vi "Generate GUID.vi"(8 "error in (no error)":errorcluster) -> (0 "error out":errorcluster, 3 "GUID":string)   [LabVIEW 2014]
panel:
  in  ".NET Refnum":refnum<k24>
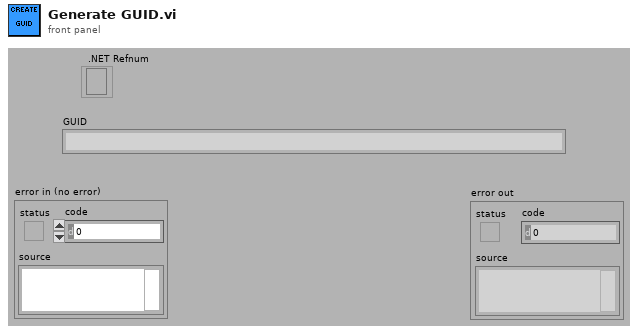
[diagram p1: front panel]
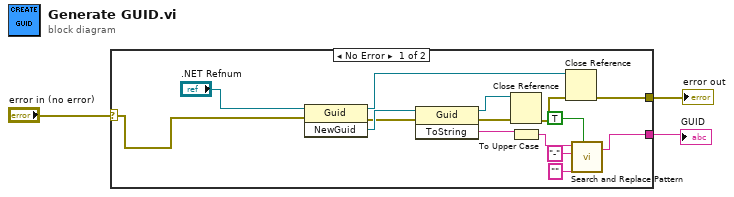
[diagram p0: block diagram]
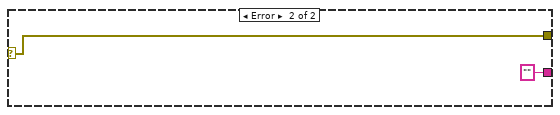
[diagram p2: hidden frame]
diagram:
  n1 = case shown="No Error" "error in (no error)" {
    selector: "error in (no error)" -> [w4 w20]
    tunnel: [w14 w20] -> w2
    tunnel: [w7 ""] -> w1
    frame No Error {
      n2 = invoke class="Guid" method="NewGuid"(reference=".NET Refnum", error in=w4) -> (reference out=w13:refnum<k24>, error out=w17:errorcluster, "NewGuid"=w18:refnum<k24>)  [unwired: 1 in]
      n3 = invoke class="Guid" method="ToString"(reference=w18, error in=w17) -> (reference out=w12:refnum<k24>, error out=w16:errorcluster, "ToString"=w11:string)  [unwired: 1 in]
      n4 = Close Reference(reference=w12, error in (no error)=w16) -> (error out=w15:errorcluster)
      n5 = To Upper Case(1:w11) -> (0:w10:string)
      n6 = Close Reference(reference=w13, error in (no error)=w15) -> (error out=w14:errorcluster)
      n7 = call <vilib>:"Search and Replace Pattern.vi"("string"=w10, "regular expression (\"\")"="-" ("regular expression (\"\")"), "replace string (\"\")"="" ("replace string (\"\")"), "replace all? (F)"=TRUE) -> ("result string"=w7:string)  [unwired: 1 in, 1 out]
    }
    frame Error {
    }
  }
  "error out" <- w2
  "GUID" <- w1
